vi "update log message.vi"(8 "error in (no error)":errorcluster, 10 "Message":string, 11 "Queue Data in":T1) -> (0 "error out":errorcluster, 3 "Queue data out":T1)   [LabVIEW 2018]
uses:
  CORE/QMH Template/Type Defs/EventsAndQueues--cluster.ctl
  CORE/Queue Messaging/Type Defs/Queue Message--cluster.ctl
  CORE/Event Messaging/Type Defs/Event Message--cluster.ctl
  CORE/Event Messaging/Event Messaging.lvlib
  CORE/Queue Messaging/Queue Messaging.lvlib
  CORE/QMH/QMH CORE.lvlib
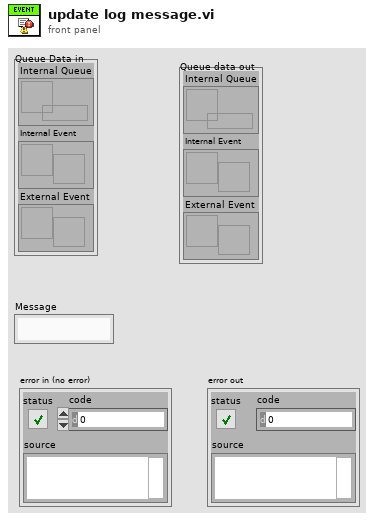
[diagram p1: front panel]
types:
  T1 = typedef "QMH CORE.lvlib/EventsAndQueues--cluster.ctl" = cluster{"Internal Queue":refnum<queue>, "Internal Event":refnum<user-event>, "External Event":refnum<user-event>}
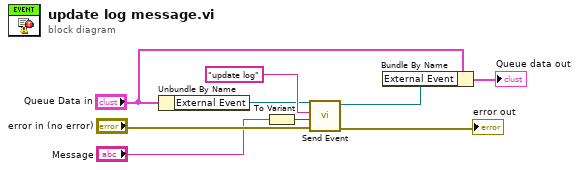
[diagram p0: block diagram]
diagram:
  n1 = Unbundle By Name("Queue Data in") -> ("External Event"=w5:refnum<user-event>)
  n2 = To Variant(anything="Message") -> (Variant=w4:variant)
  n3 = call "Send Event.vi"("Error in"="error in (no error)", "Data"=w4, "Cmd"="update log", "Event Ref"=w5) -> ("Error out"=→"error out":errorcluster, "Event Ref out"=w3:refnum<user-event>)  [unwired: 6 in]
  n4 = Bundle By Name(cluster="Queue Data in", "External Event"=w3) -> (→"Queue data out":T1)
